vi "shift test.vi"() -> ()   [LabVIEW 2020]
uses:
  <vilib>/rvi/FXPMathLib/FxpInterpret/XNode/nifxpmath_Interpret.xnode
panel:
  out "y":fxp<+,8,7>
  in  "x":fxp<+,8,0>
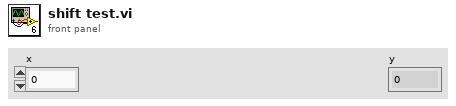
[diagram p1: front panel]
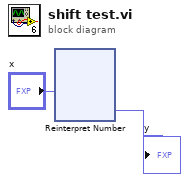
[diagram p0: block diagram]
diagram:
  n1 = xnode "Reinterpret Number"("x"="x") -> ("y"=→"y":fxp<+,8,7>)
